vi "Init I2C.vi"(4 "SDA GPIO":T2=-1, 5 "Pullup (F)":bool, 6 "SCL GPIO":T2=-1, 7 "I2C #":T1=-1, 8 "error in (no error)":errorcluster, 10 "Baud":u32=400000 format="%.0p", 11 "VisaSession in":refnum<class "VisaSession.lvclass">) -> (0 "error out":errorcluster, 2 "I2C":refnum<class "I2C.lvclass">, 3 "VisaSession out":refnum<class "VisaSession.lvclass">)   [LabVIEW 2020, in "CTI.lvlib" / "VisaSession.lvclass"]
uses:
  VisaSession.lvclass
  VisaSession.lvclass/VisaSession.ctl
  Session/Session.lvclass
  GPIO Number.ctl
  CTI.lvlib
  I2C Number.ctl
  I2C/I2C.lvclass
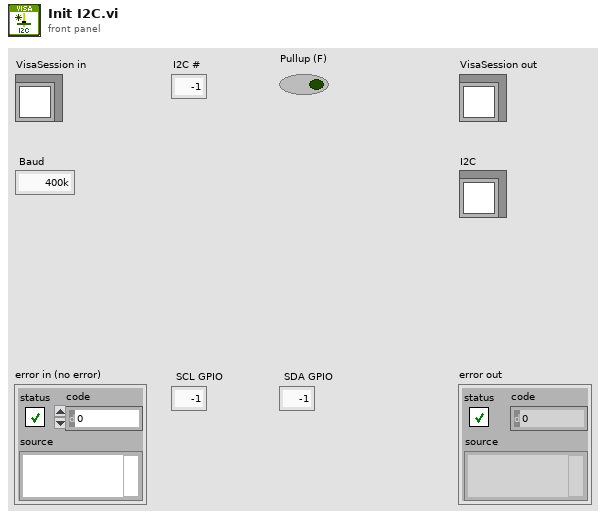
[diagram p1: front panel]
types:
  T1 = typedef "CTI.lvlib/I2C Number.ctl" = i8
  T2 = typedef "CTI.lvlib/GPIO Number.ctl" = i8
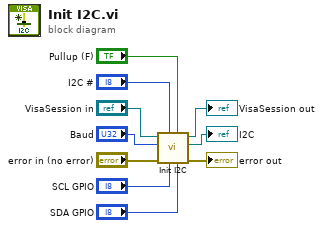
[diagram p0: block diagram]
diagram:
  n1 = call-parent "Init I2C.vi"("SDA GPIO"="SDA GPIO", "Pullup (F)"="Pullup (F)", "SCL GPIO"="SCL GPIO", "I2C #"="I2C #", "error in (no error)"="error in (no error)", "Baud"="Baud", "Session in"="VisaSession in") -> ("error out"=→"error out":errorcluster, "I2C"=→"I2C":refnum<class "I2C.lvclass">, "Session out"=→"VisaSession out":refnum<class "VisaSession.lvclass">)  [unwired: 2 in]
